vi "SwitchBoard_test.vi"() -> ()   [LabVIEW 2016]
panel:
  out "error out":errorcluster
  out "Current channel":i32
  out "Hum":string
  out "Temp":string
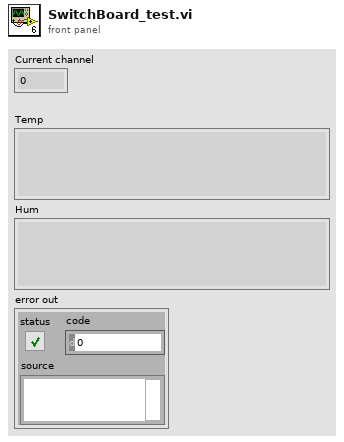
[diagram p1: front panel]
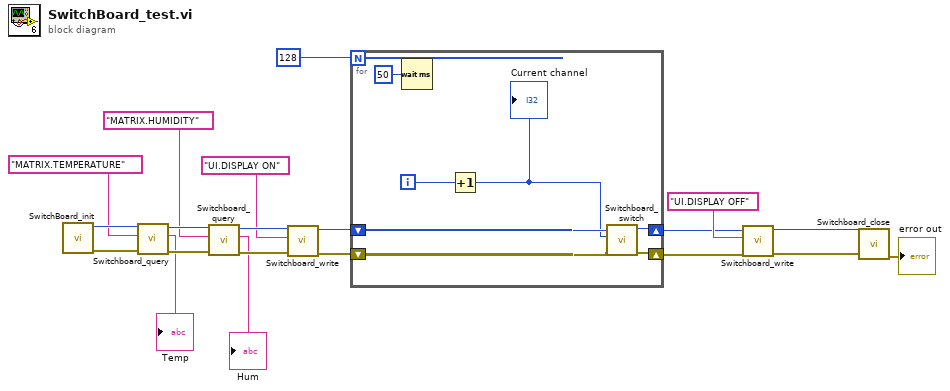
[diagram p0: block diagram]
diagram:
  n1 = call "SwitchBoard_init.vi"() -> ("error out"=w20:errorcluster, "Handle"=w16:u32)  [unwired: 10 in]
  n2 = call "Switchboard_query.vi"("error in"=w20, "Buffer"="MATRIX.TEMPERATURE", "Handle"=w16) -> ("error out"=w19:errorcluster, "Read Buffer Out"=→"Temp":string, "Handle"=w15:u32)  [unwired: 6 in]
  n3 = call "Switchboard_query.vi"("error in"=w19, "Buffer"="MATRIX.HUMIDITY", "Handle"=w15) -> ("error out"=w18:errorcluster, "Read Buffer Out"=→"Hum":string, "Handle"=w14:u32)  [unwired: 6 in]
  n4 = call "Switchboard_write.vi"("error in"=w18, "Buffer"="UI.DISPLAY ON", "Handle"=w14) -> ("error out"=w17:errorcluster, "Handle"=w13:u32)  [unwired: 7 in]
  n5 = for {
    N: 128 -> [_]
    shift-right: [w24] -> w4
    shift-left: w17 -> [w23]
    shift-right: [w25] -> w2
    shift-left: w13 -> [w22]
    i -> [w27]
    n6 = Wait (ms)(milliseconds to wait=u32 50) -> ()  [unwired: 1 out]
    n7 = Increment(x=w27) -> (x+1=w21:i32)
    "Current channel" <- w21
    n8 = call "Switchboard_switch.vi"("error in"=w23, "Channel"=w21, "Handle"=w22) -> ("error out"=w24:errorcluster, "Handle"=w25:u32)  [unwired: 7 in]
  }
  n9 = call "Switchboard_write.vi"("error in"=w4, "Buffer"="UI.DISPLAY OFF", "Handle"=w2) -> ("error out"=w3:errorcluster, "Handle"=w1:u32)  [unwired: 7 in]
  n10 = call "Switchboard_close.vi"("error in"=w3, "Handle"=w1) -> ("error out"=→"error out":errorcluster)  [unwired: 8 in, 1 out]
